vi "demo_create.vi"() -> ()   [LabVIEW 2021]
panel:
  in  "Tree":string(tree)
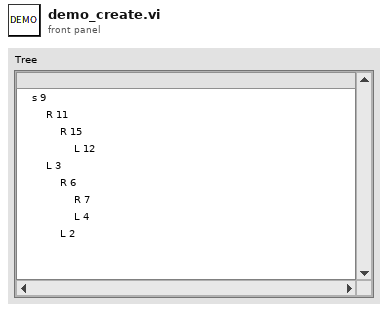
[diagram p1: front panel]
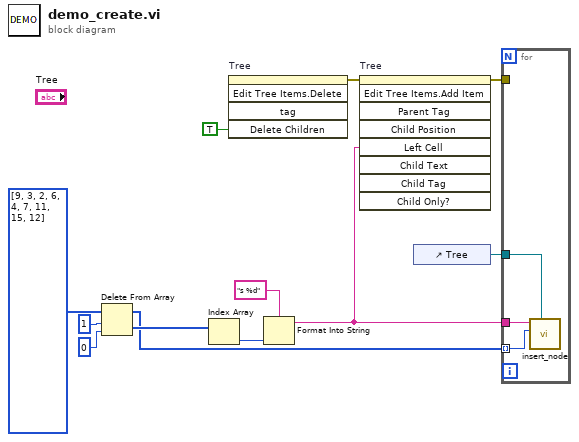
[diagram p0: block diagram]
diagram:
  n1 = Delete From Array "Delete From Array"(array=i32[] [9, 3, 2, 6, 4, 7, 11, 15, 12], length=1, index=0) -> (deleted portion=w6:i32[], array with subset deleted=w4:i32[])
  n2 = Index Array(array=w6) -> (element=w11:i32)  [unwired: 1 in]
  n3 = invoke on="Tree" class="Tree (strict)" method="Edit Tree Items.Delete"("Delete Children"=TRUE ("Delete Children?")) -> (error out=w9:errorcluster)  [unwired: 4 in, 4 out]
  n4 = Format Into String(format string="s %d", w11) -> (resulting string=w3:string)  [unwired: 2 in, 1 out]
  n5 = invoke on="Tree" class="Tree (strict)" method="Edit Tree Items.Add Item"(error in=w9, "Left Cell"=w3) -> (error out=w1:errorcluster)  [unwired: 7 in, 8 out]
  n6 = control-ref of="Tree"() -> (w2:refnum<vi>)
  n7 = for {
    tunnel: w4 -> [w15] mode=indexing
    tunnel: w3 -> [w14]
    tunnel: w2 -> [w13]
    tunnel: w1 -> [_]
    n8 = call "insert_node.vi"("tree"=w13, "value"=w15, "node"=w14) -> ()  [unwired: 9 in]
  }
